vi "Connect.vi"(6 "Access":T1, 8 "error in (no error)":errorcluster, 11 "PVConnection in":refnum<class "SVConnection.lvclass">) -> (0 "error out":errorcluster, 3 "PVConnection out":refnum<class "SVConnection.lvclass">)   [LabVIEW 2012, in "CS++ProcessVariables.lvlib" / "SVConnection.lvclass"]
doc: "Opene reference to a shared variable if not already connected."
uses:
  SVConnection.lvclass
  SVConnection.lvclass/SVConnection.ctl
  PVConnection/PVConnection.lvclass/PVConnection.ctl
  PVConnection/PVConnection.lvclass
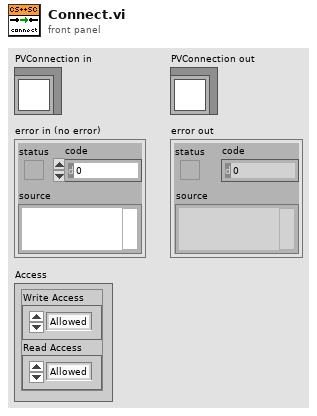
[diagram p1: front panel]
types:
  T1 = cluster{"Write Access":enum8{"Allowed", "Required", "None"}, "Read Access":enum8{"Allowed", "Required", "None"}}
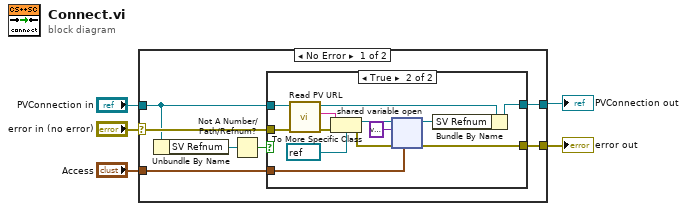
[diagram p0: block diagram]
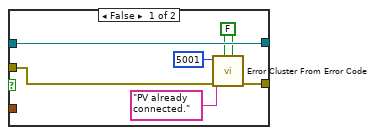
[diagram p2: hidden frame]
diagram:
  n1 = case shown="No Error" "error in (no error)" {
    selector: "error in (no error)" -> [w12 w33]
    tunnel: [w11 w33] -> w4
    tunnel: [w10 w32] -> w2
    tunnel: "PVConnection in" -> [w9 w32]
    tunnel: "Access" -> [w6 _]
    frame No Error {
      n2 = Unbundle By Name(w9) -> ("SV Refnum"=w8:refnum<k21>)
      n3 = Not A Number/Path/Refnum?(number/path/refnum=w8) -> (NaN/Path/Refnum?=w7:bool)
      n4 = case shown="True" w7 {
        tunnel: w12 -> [w17 w25]
        tunnel: [w16 w24] -> w11
        tunnel: [w18 w21] -> w10
        tunnel: w9 -> [w18 w20]
        tunnel: w6 -> [_ w19]
        frame False {
          w15 = FALSE ("show call chain? (False)")
          n5 = call <vilib>:"Error Cluster From Error Code.vi"("is warning? (False)"=w15, "show call chain? (False)"=w15, "error in (no error)"=w17, "error message (\"\")"="PV already connected." ("error message (\"\")"), "error code (0)"=5001) -> ("error out"=w16:errorcluster)  [unwired: 4 in]
        }
        frame True {
          n6 = call "Read PV URL.vi"("error in (no error)"=w25, "PVConnection in"=w20) -> ("error out"=w29:errorcluster, "PV URL"=w31:string, "PVConnection out"=w22:refnum<class "SVConnection.lvclass">)  [unwired: 7 in]
          n7 = To More Specific Class(target class=refnum<k21> refnum ("shared variable refnum in"), reference=w31, error in=w29) -> (specific class reference=w28:refnum<k21>, error out=w27:errorcluster)
          n8 = shared-variable-open(w28, w27, variant ("variant"), w19) -> (w23:refnum<k21>, w24:errorcluster)
          n9 = Bundle By Name(cluster=w22, "SV Refnum"=w23) -> (w21:refnum<class "SVConnection.lvclass">)
        }
      }
    }
    frame Error {
    }
  }
  "error out" <- w4
  "PVConnection out" <- w2
